vi "Insert Multiple Events(Error).vi"(6 "Insert Selected?":bool[](array[boolean]), 8 "error in (no error)":errorcluster, 9 "Insert all? (T)":bool=TRUE, 10 "Events to Insert":string[](array[string]), 11 "Event queue in":string[](array[string])) -> (0 "error out":errorcluster, 3 "Event queue out":string[](array[string]))   [LabVIEW 2014]
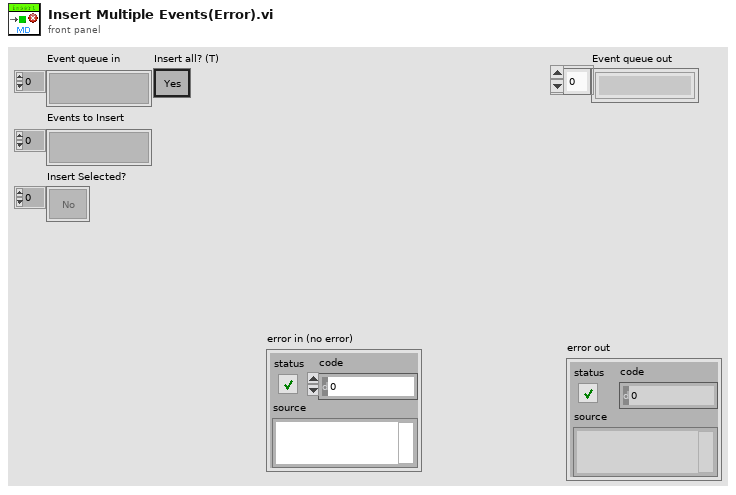
[diagram p1: front panel]
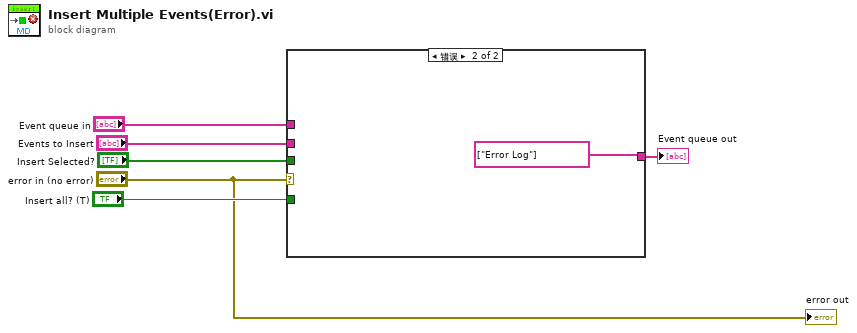
[diagram p0: block diagram]
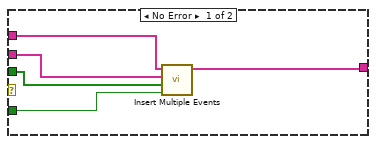
[diagram p2: hidden frame]
diagram:
  n1 = case shown="错误" "error in (no error)" {
    tunnel: "Insert all? (T)" -> [w11 _]
    tunnel: "Insert Selected?" -> [w10 _]
    tunnel: "Events to Insert" -> [w9 _]
    tunnel: "Event queue in" -> [w8 _]
    tunnel: [w7 string[] ["Error Log"]] -> w1
    frame No Error {
      n2 = call "Insert Multiple Events.vi"("Insert all? (T)"=w11, "Insert Selected?"=w10, "Events to Insert"=w9, "Event queue in"=w8) -> ("Event queue out"=w7:string[])  [unwired: 3 in]
    }
    frame Error {
    }
  }
  "Event queue out" <- w1
  "error out" <- "error in (no error)"
